vi "Display Tree & Create Node Values.vi"(8 "error in (no error)":errorcluster, 10 "Linked Nodes IN":T1[](array[typedef]), 11 "TreeControl in":refnum<vi>) -> (0 "error out":errorcluster, 2 "Nodes values":string[][](array[string]), 3 "TreeControl OUT":refnum<vi>)   [LabVIEW 2017]
uses:
  BinaryNode.ctl
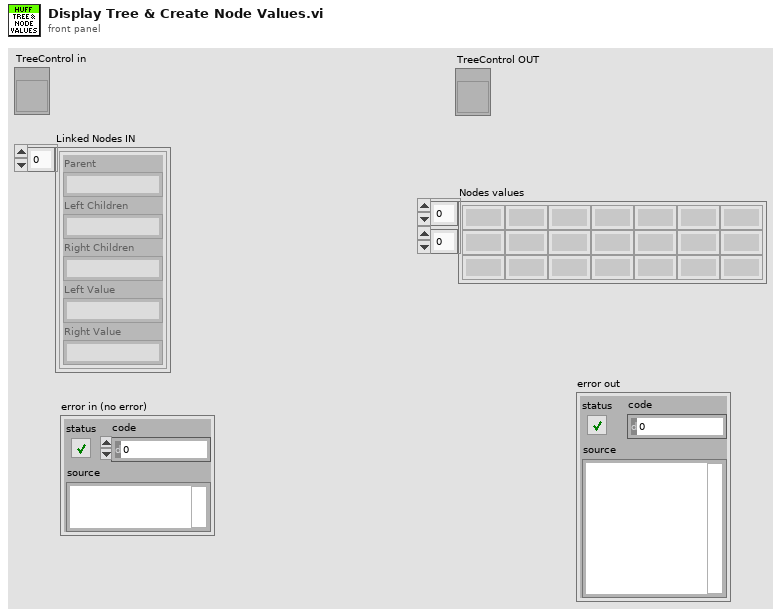
[diagram p1: front panel]
types:
  T1 = typedef "BinaryNode.ctl" = cluster{"Parent":string, "Left Children":string, "Right Children":string, "Left Value":string, "Right Value":string}
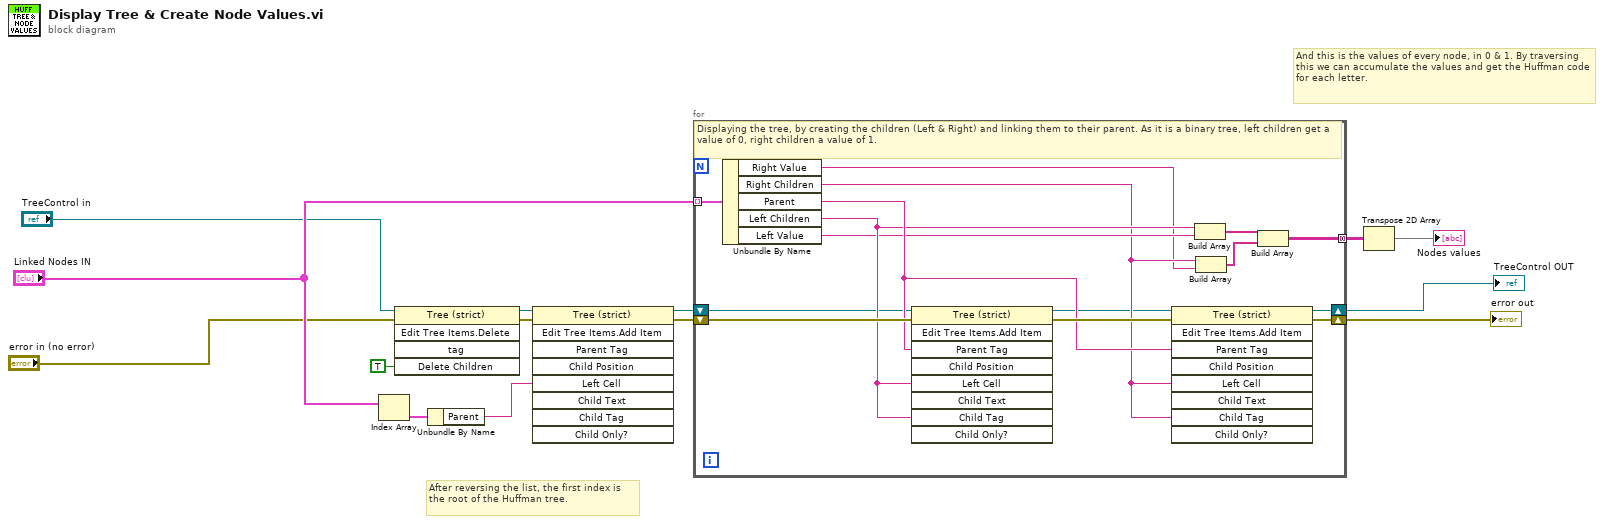
[diagram p0: block diagram]
diagram:
  # "And this is the values of every node, in 0 & 1. By traversing this we can accumulate the values and get the Huffman code for each letter."
  # "After reversing the list, the first index is the root of the Huffman tree."
  n1 = Index Array(array="Linked Nodes IN") -> (element=w6:T1)  [unwired: 1 in]
  n2 = invoke on="Invoke Node" class="Tree (strict)" method="Edit Tree Items.Delete"(reference="TreeControl in", error in="error in (no error)", "Delete Children"=TRUE ("Delete Children?")) -> (reference out=w2:refnum<vi>, error out=w8:errorcluster)  [unwired: 2 in, 3 out]
  n3 = Unbundle By Name(w6) -> ("Parent"=w10:string)
  n4 = invoke on="Invoke Node" class="Tree (strict)" method="Edit Tree Items.Add Item"(reference=w2, error in=w8, "Left Cell"=w10) -> (reference out=w4:refnum<vi>, error out=w7:errorcluster)  [unwired: 6 in, 7 out]
  n5 = for {
    tunnel: "Linked Nodes IN" -> [w26] mode=indexing
    shift-right: [w27] -> w11
    shift-left: w7 -> [w29]
    tunnel: [w18] -> w12 mode=concatenating
    shift-right: [w15] -> w3
    shift-left: w4 -> [w17]
    # "Displaying the tree, by creating the children (Left & Right) and linking them to their parent. As it is a binary tree, left children get a value of 0, right children a value of 1."
    n6 = Unbundle By Name(w26) -> ("Right Value"=w19:string, "Right Children"=w20:string, "Parent"=w25:string, "Left Children"=w22:string, "Left Value"=w21:string)
    n7 = invoke on="Invoke Node" class="Tree (strict)" method="Edit Tree Items.Add Item"(reference=w17, error in=w29, "Parent Tag"=w25, "Left Cell"=w22, "Child Tag"=w22) -> (reference out=w16:refnum<vi>, error out=w28:errorcluster)  [unwired: 4 in, 7 out]
    n8 = invoke on="Invoke Node" class="Tree (strict)" method="Edit Tree Items.Add Item"(reference=w16, error in=w28, "Parent Tag"=w25, "Left Cell"=w20, "Child Tag"=w20) -> (reference out=w15:refnum<vi>, error out=w27:errorcluster)  [unwired: 4 in, 7 out]
    n9 = Build Array(w22, w21) -> (w24:string[])
    n10 = Build Array(w20, w19) -> (w23:string[])
    n11 = Build Array(w24, w23) -> (w18:string[][])
  }
  "error out" <- w11
  "TreeControl OUT" <- w3
  n12 = Transpose 2D Array(2D array=w12) -> (transposed array=→"Nodes values":string[][])
